vi "报告打印.vi"(9 "输出簇":T1, 11 "打印?":bool) -> ()   [LabVIEW 2010]
uses:
  <vilib>/Utility/NIReport.llb/NI_report.lvclass
  <vilib>/Utility/NIReport.llb/Append Report Text (str wrap).vi
  全局量/试验配置信息.vi
  <vilib>/addons/_office/word.llb/Word Easy Table (str).vi
  <vilib>/addons/_office/NI_ReportGenerationToolkit.lvlib
panel:
  in  "序号":i32
  out "XY图":cluster{"Y":dbl[], "Y":dbl[]}[](graph)
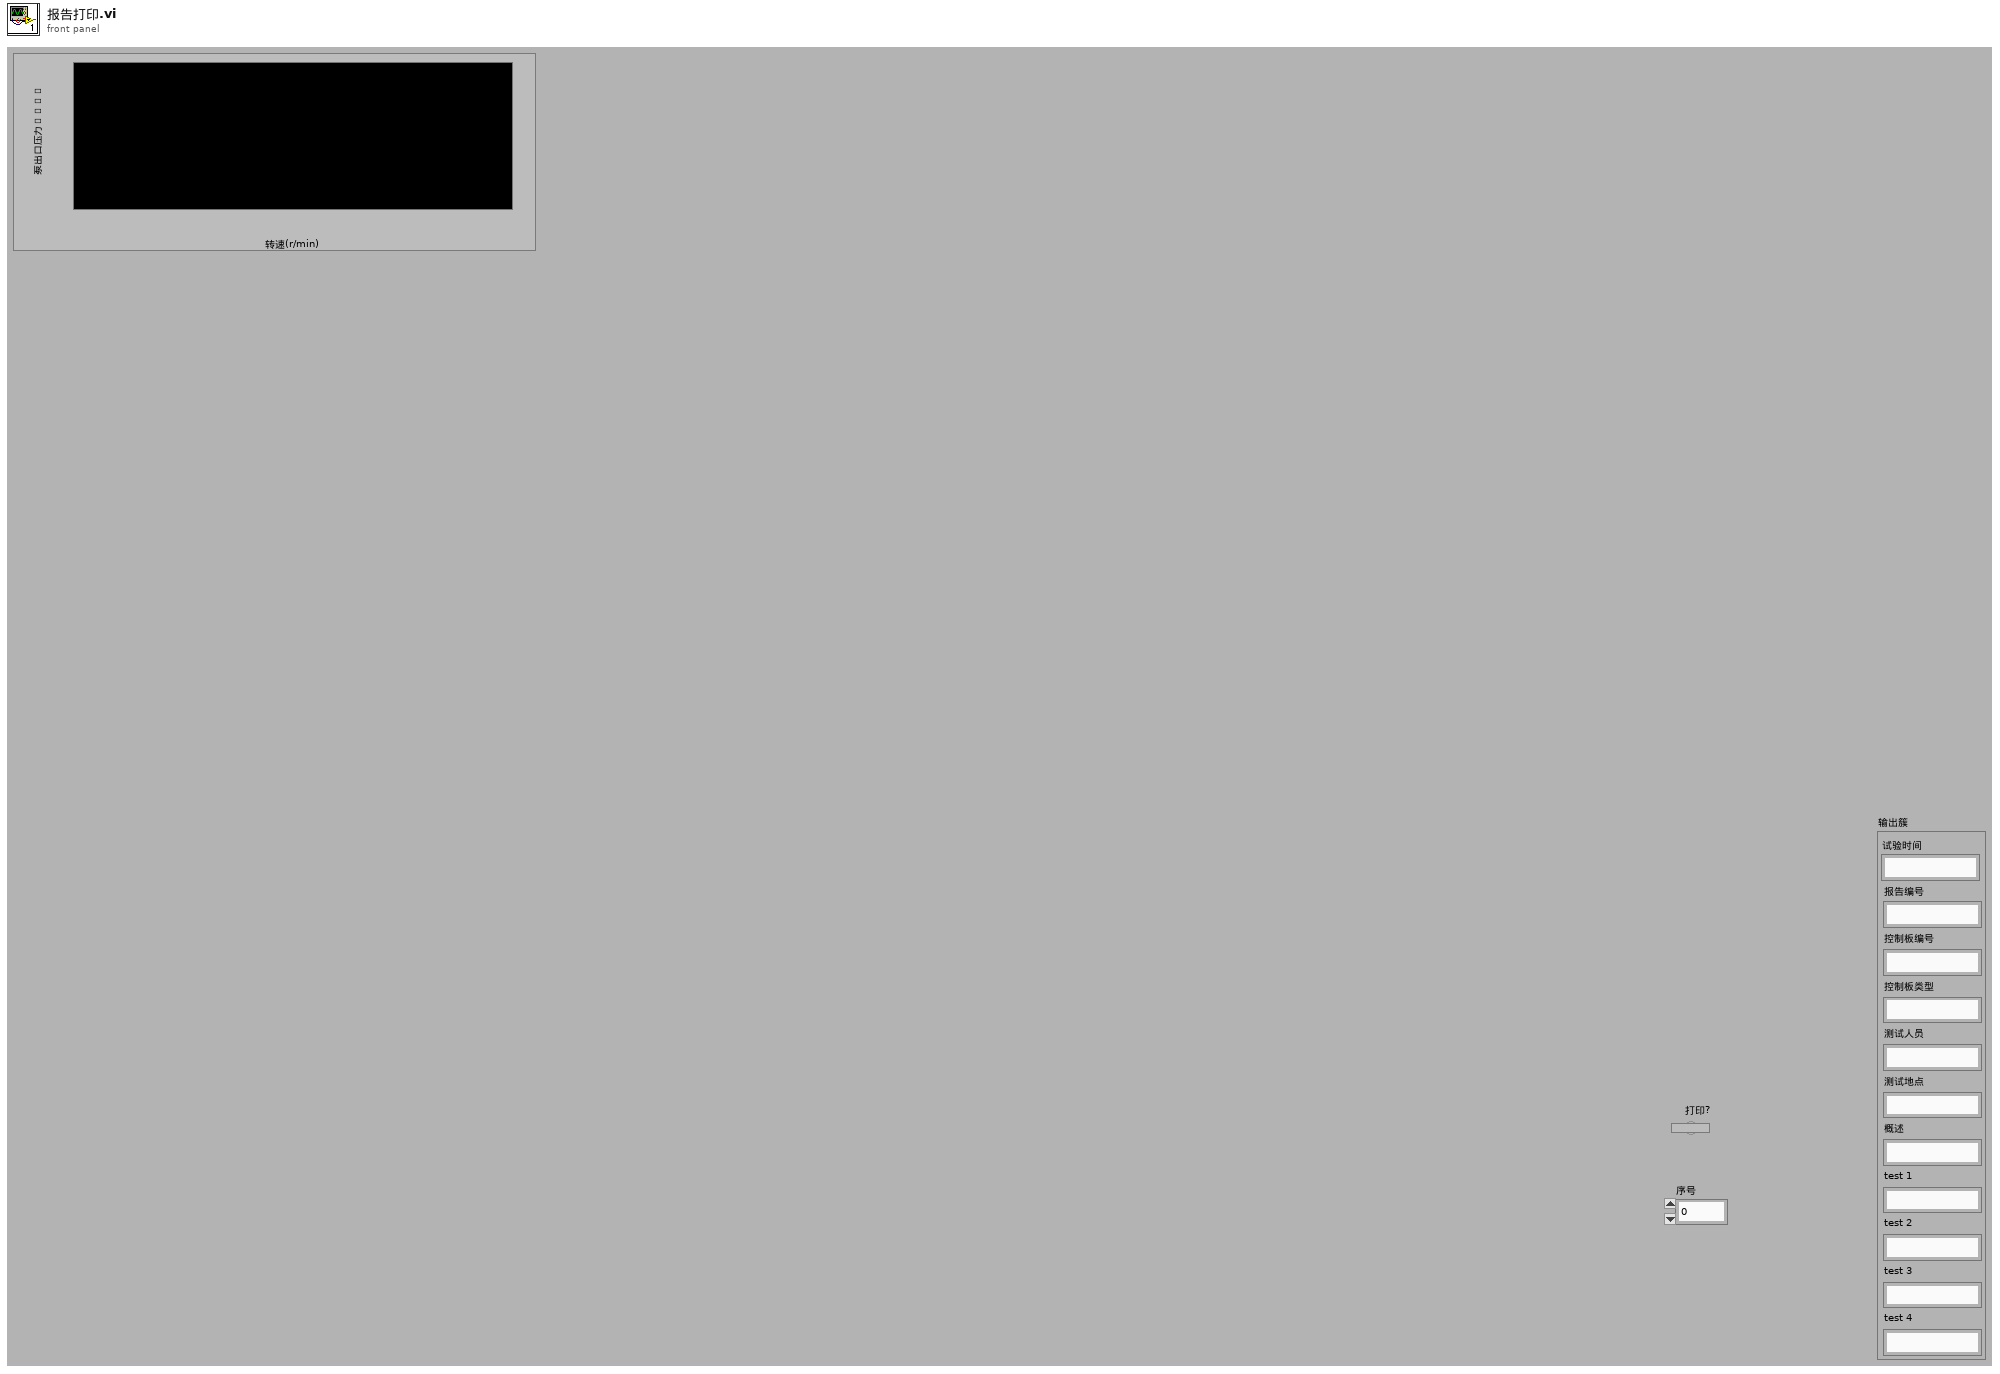
[diagram p1: front panel]
types:
  T1 = cluster{"试验时间":string, "报告编号":string, "控制板编号":string, "控制板类型":string, "测试人员":string, "测试地点":string, "概述":string, "test 1":string, "test 2":string, "test 3":string, "test 4":string}
  T2 = cluster{"position (Excel)":cluster{"row":i32, "column":i32}, "name (Excel)":string, "bookmark (Word)":string}
  T3 = enum16{"maximized", "minimized", "normal", "no change"}
  T4 = enum16{"Standard Report", "HTML", "Word", "Excel"}
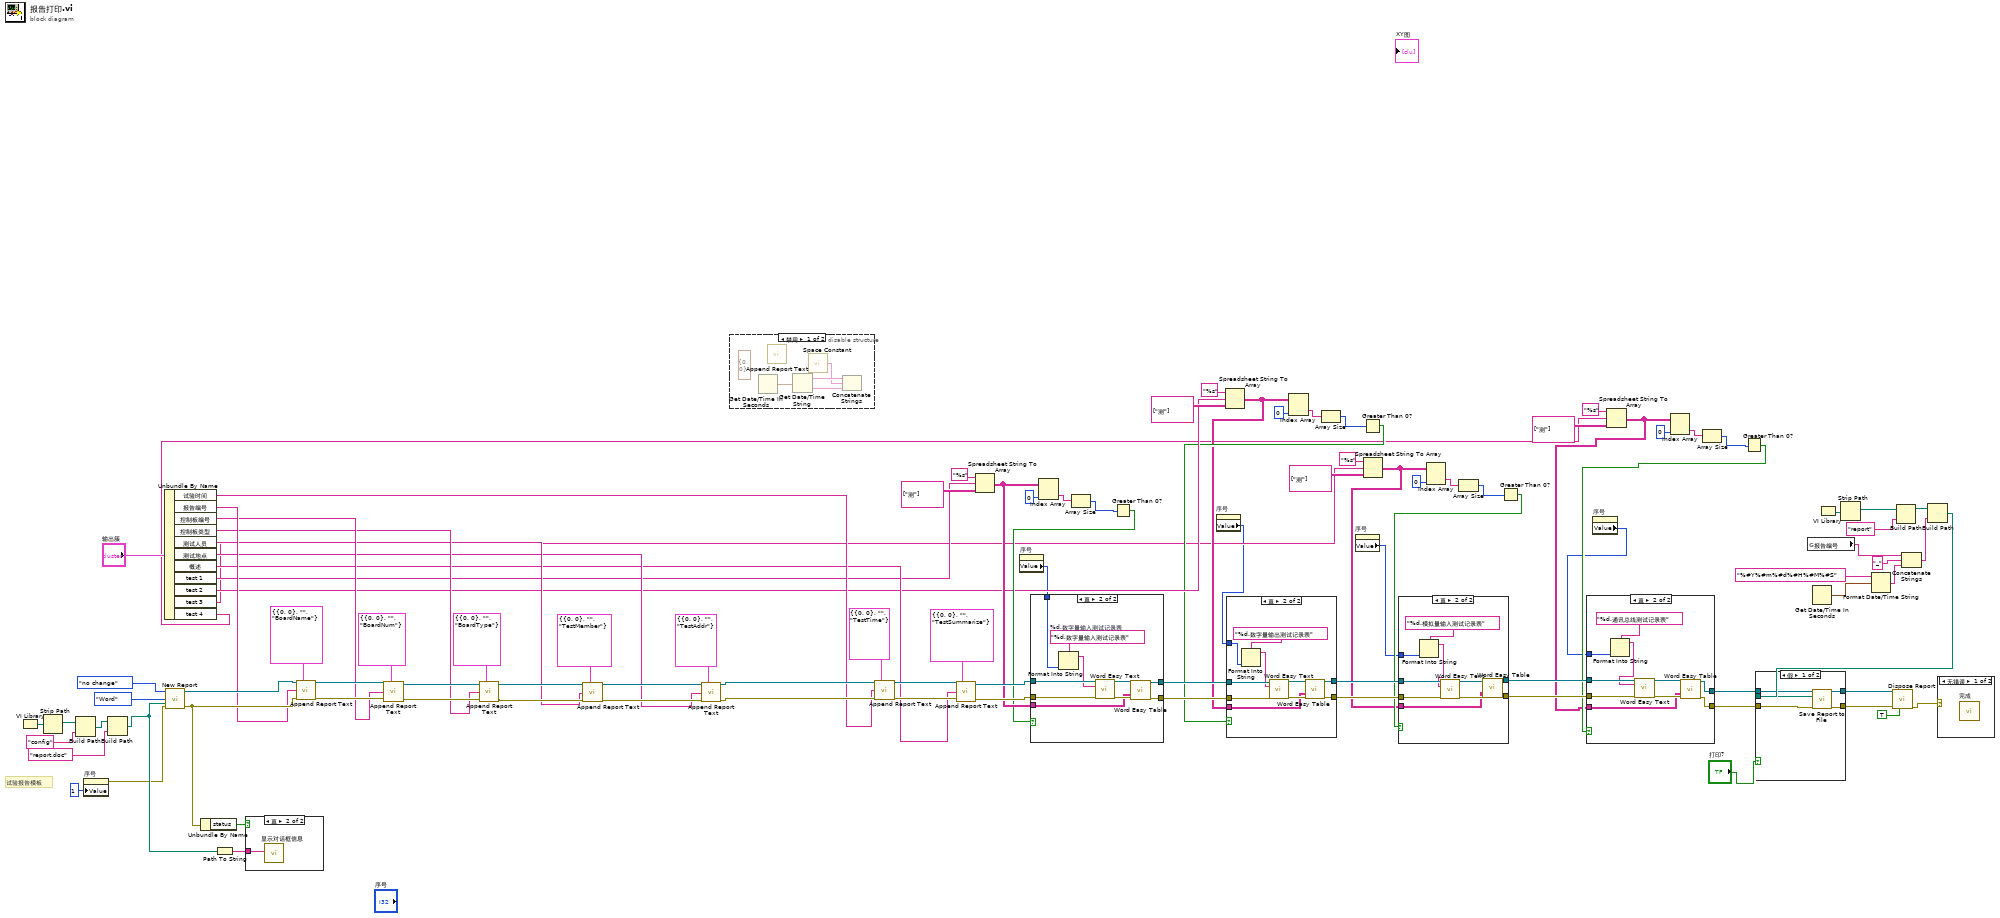
[diagram p0: block diagram]
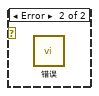
[diagram p6: hidden frame]
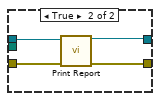
[diagram p7: hidden frame]
diagram:
  # "试验报告模板"
  n1 = VI Library() -> (path=w97:path)
  n2 = Strip Path(path=w97) -> (stripped path=w94:path)  [unwired: 1 out]
  n3 = Build Path(base path=w94, name or relative path="config") -> (appended path=w96:path)
  n4 = property on="序号" class="DigNum (严格)"("Value"=1 ("序号")) -> (error out=w49:errorcluster)  [unwired: 2 in, 1 out]
  n5 = Build Path(base path=w96, name or relative path="report.doc") -> (appended path=w100:path)
  n6 = Unbundle By Name("输出簇") -> ("试验时间"=w39:string, "报告编号"=w44:string, "控制板编号"=w43:string, "控制板类型"=w42:string, "测试人员"=w41:string, "测试地点"=w40:string, "概述"=w38:string, "test 1"=w35:string, "test 2"=w25:string, "test 3"=w18:string, "test 4"=w11:string)
  n7 = call <vilib>:"New Report.vi"("window state (normal)"=T3."no change", "report type"=T4."Word", "template (empty)"=w100, "error in (no error)"=w49) -> ("report out"=w91:refnum<class "NI_report.lvclass">, "error out"=w90:errorcluster)  [unwired: 10 in]
  n8 = Unbundle By Name(w90) -> ("status"=w102:bool)
  n9 = Path To String(path=w100) -> (string=w101:string)
  n10 = case shown="真" w102 {
    tunnel: w101 -> [_ w104]
    frame False {
    }
    frame True {
      n11 = call "显示对话框信息"("Message"=w104) -> ()  [unwired: 9 in, 2 out]
    }
  }
  n12 = call-poly <vilib>:"Append Report Text.vi"("report in"=w91, "MS Office parameters"=T2 {"position (Excel)"={"row"=0, "column"=0}, "name (Excel)"="", "bookmark (Word)"="BoardName"}, "text"=w44, "error in (no error)"=w90) -> ("report out"=w76:refnum<class "NI_report.lvclass">, "error out"=w75:errorcluster)  [unwired: 8 in, 2 out]
  n13 = call-poly <vilib>:"Append Report Text.vi"("report in"=w76, "MS Office parameters"=T2 {"position (Excel)"={"row"=0, "column"=0}, "name (Excel)"="", "bookmark (Word)"="BoardNum"}, "text"=w43, "error in (no error)"=w75) -> ("report out"=w86:refnum<class "NI_report.lvclass">, "error out"=w85:errorcluster)  [unwired: 8 in, 2 out]
  n14 = call-poly <vilib>:"Append Report Text.vi"("report in"=w86, "MS Office parameters"=T2 {"position (Excel)"={"row"=0, "column"=0}, "name (Excel)"="", "bookmark (Word)"="BoardType"}, "text"=w42, "error in (no error)"=w85) -> ("report out"=w83:refnum<class "NI_report.lvclass">, "error out"=w82:errorcluster)  [unwired: 8 in, 2 out]
  n15 = call-poly <vilib>:"Append Report Text.vi"("report in"=w83, "MS Office parameters"=T2 {"position (Excel)"={"row"=0, "column"=0}, "name (Excel)"="", "bookmark (Word)"="TestMember"}, "text"=w41, "error in (no error)"=w82) -> ("report out"=w80:refnum<class "NI_report.lvclass">, "error out"=w79:errorcluster)  [unwired: 8 in, 2 out]
  n16 = call-poly <vilib>:"Append Report Text.vi"("report in"=w80, "MS Office parameters"=T2 {"position (Excel)"={"row"=0, "column"=0}, "name (Excel)"="", "bookmark (Word)"="TestAddr"}, "text"=w40, "error in (no error)"=w79) -> ("report out"=w78:refnum<class "NI_report.lvclass">, "error out"=w77:errorcluster)  [unwired: 8 in, 2 out]
  n17 = disable-structure shown="禁用" {
    frame Disabled {
      (unwired) cluster{"row":i32, "column":i32} {"row"=0, "column"=0} ("position (excel)")
      n18 = Get Date/Time In Seconds() -> (seconds since 1Jan1904=w108:timestamp)
      n19 = call-poly <vilib>:"Append Report Text.vi"() -> ()  [unwired: 12 in, 4 out]
      n20 = Get Date/Time String(seconds (now)=w108) -> (date string=w107:string, time string=w106:string)  [unwired: 2 in]
      n21 = call <vilib>:"Space Constant.vi"() -> ("String"=w105:string)
      n22 = Concatenate Strings(w107, w105, w106) -> ()  [unwired: 1 out]
    }
    frame Enabled {
    }
  }
  n23 = call-poly <vilib>:"Append Report Text.vi"("report in"=w78, "MS Office parameters"=T2 {"position (Excel)"={"row"=0, "column"=0}, "name (Excel)"="", "bookmark (Word)"="TestTime"}, "text"=w39, "error in (no error)"=w77) -> ("report out"=w54:refnum<class "NI_report.lvclass">, "error out"=w53:errorcluster)  [unwired: 8 in, 2 out]
  n24 = call-poly <vilib>:"Append Report Text.vi"("report in"=w54, "MS Office parameters"=T2 {"position (Excel)"={"row"=0, "column"=0}, "name (Excel)"="", "bookmark (Word)"="TestSummarize"}, "text"=w38, "error in (no error)"=w53) -> ("report out"=w52:refnum<class "NI_report.lvclass">, "error out"=w51:errorcluster)  [unwired: 8 in, 2 out]
  n25 = Spreadsheet String To Array(format string="%s" ("格式字符串"), spreadsheet string=w35, array type (2D Dbl)=string[][] [["测"]] ("数组类型(2D String)")) -> (array=w34:string[][])  [unwired: 1 in]
  n26 = property on="序号" class="DigNum (严格)"() -> ("Value"=w7:i32)  [unwired: 2 in, 2 out]
  n27 = Index Array(array=w34, index (col)=0 ("禁用的索引 (列)")) -> (element=w32:string[])  [unwired: 1 in]
  n28 = Array Size(array=w32) -> (size(s)=w31:i32)
  n29 = Greater Than 0?(x=w31) -> (x > 0?=w30:bool)
  n30 = case shown="真" w30 {
    tunnel: [w110 w119] -> w61
    tunnel: [w109 w118] -> w59
    tunnel: w52 -> [w110 w116]
    tunnel: w51 -> [w109 w115]
    tunnel: w34 -> [_ w112]
    tunnel: w7 -> [_ w111]
    frame False {
    }
    frame True {
      w114 = "%d.数字量输入测试记录表"  # %d.数字量输入测试记录表
      n31 = Format Into String(format string=w114, w111) -> (resulting string=w113:string)  [unwired: 2 in, 1 out]
      n32 = call <vilib>:"Word Easy Text.vi"("report in"=w116, "text"=w113, "error in (no error)"=w115) -> ("report out"=w120:refnum<class "NI_report.lvclass">, "error out"=w117:errorcluster)  [unwired: 10 in, 1 out]
      n33 = call-poly <vilib>:"Word Easy Table.vi"("report in"=w120, "data"=w112, "error in (no error)"=w117) -> ("report out"=w119:refnum<class "NI_report.lvclass">, "error out"=w118:errorcluster)  [unwired: 10 in, 1 out]
    }
  }
  n34 = property on="序号" class="DigNum (严格)"() -> ("Value"=w6:i32)  [unwired: 2 in, 2 out]
  n35 = Spreadsheet String To Array(format string="%s" ("格式字符串"), spreadsheet string=w25, array type (2D Dbl)=string[][] [["测"]] ("数组类型(2D String)")) -> (array=w23:string[][])  [unwired: 1 in]
  n36 = Index Array(array=w23, index (col)=0 ("禁用的索引 (列)")) -> (element=w26:string[])  [unwired: 1 in]
  n37 = Array Size(array=w26) -> (size(s)=w5:i32)
  n38 = property on="序号" class="DigNum (严格)"() -> ("Value"=w4:i32)  [unwired: 2 in, 2 out]
  n39 = Greater Than 0?(x=w5) -> (x > 0?=w24:bool)
  n40 = case shown="真" w24 {
    tunnel: w61 -> [w122 w132]
    tunnel: [w122 w130] -> w60
    tunnel: w59 -> [w121 w129]
    tunnel: [w121 w127] -> w58
    tunnel: w6 -> [_ w124]
    tunnel: w23 -> [_ w123]
    frame False {
    }
    frame True {
      n41 = Format Into String(format string="%d.数字量输出测试记录表", w124) -> (resulting string=w125:string)  [unwired: 2 in, 1 out]
      n42 = call <vilib>:"Word Easy Text.vi"("report in"=w132, "text"=w125, "error in (no error)"=w129) -> ("report out"=w131:refnum<class "NI_report.lvclass">, "error out"=w128:errorcluster)  [unwired: 10 in, 1 out]
      n43 = call-poly <vilib>:"Word Easy Table.vi"("report in"=w131, "data"=w123, "error in (no error)"=w128) -> ("report out"=w130:refnum<class "NI_report.lvclass">, "error out"=w127:errorcluster)  [unwired: 10 in, 1 out]
    }
  }
  n44 = Spreadsheet String To Array(format string="%s" ("格式字符串"), spreadsheet string=w18, array type (2D Dbl)=string[][] [["测"]] ("数组类型(2D String)")) -> (array=w16:string[][])  [unwired: 1 in]
  n45 = Index Array(array=w16, index (col)=0 ("禁用的索引 (列)")) -> (element=w19:string[])  [unwired: 1 in]
  n46 = Array Size(array=w19) -> (size(s)=w3:i32)
  n47 = Greater Than 0?(x=w3) -> (x > 0?=w17:bool)
  n48 = case shown="真" w17 {
    tunnel: w60 -> [w134 w144]
    tunnel: w58 -> [w133 w142]
    tunnel: [w134 w140] -> w57
    tunnel: [w133 w139] -> w56
    tunnel: w4 -> [_ w136]
    tunnel: w16 -> [_ w135]
    frame False {
    }
    frame True {
      n49 = Format Into String(format string="%d.模拟量输入测试记录表", w136) -> (resulting string=w137:string)  [unwired: 2 in, 1 out]
      n50 = call <vilib>:"Word Easy Text.vi"("report in"=w144, "text"=w137, "error in (no error)"=w142) -> ("report out"=w143:refnum<class "NI_report.lvclass">, "error out"=w141:errorcluster)  [unwired: 10 in, 1 out]
      n51 = call-poly <vilib>:"Word Easy Table.vi"("report in"=w143, "data"=w135, "error in (no error)"=w141) -> ("report out"=w140:refnum<class "NI_report.lvclass">, "error out"=w139:errorcluster)  [unwired: 10 in, 1 out]
    }
  }
  n52 = property on="序号" class="DigNum (严格)"() -> ("Value"=w2:i32)  [unwired: 2 in, 2 out]
  n53 = Spreadsheet String To Array(format string="%s" ("格式字符串"), spreadsheet string=w11, array type (2D Dbl)=string[][] [["测"]] ("数组类型(2D String)")) -> (array=w9:string[][])  [unwired: 1 in]
  n54 = Index Array(array=w9, index (col)=0 ("禁用的索引 (列)")) -> (element=w12:string[])  [unwired: 1 in]
  n55 = Array Size(array=w12) -> (size(s)=w1:i32)
  n56 = Greater Than 0?(x=w1) -> (x > 0?=w10:bool)
  n57 = case shown="真" w10 {
    tunnel: [w146 w156] -> w63
    tunnel: [w145 w155] -> w62
    tunnel: w57 -> [w146 w154]
    tunnel: w56 -> [w145 w153]
    tunnel: w2 -> [_ w148]
    tunnel: w9 -> [_ w147]
    frame False {
    }
    frame True {
      n58 = Format Into String(format string="%d.通讯总线测试记录表", w148) -> (resulting string=w149:string)  [unwired: 2 in, 1 out]
      n59 = call <vilib>:"Word Easy Text.vi"("report in"=w154, "text"=w149, "error in (no error)"=w153) -> ("report out"=w152:refnum<class "NI_report.lvclass">, "error out"=w151:errorcluster)  [unwired: 10 in, 1 out]
      n60 = call-poly <vilib>:"Word Easy Table.vi"("report in"=w152, "data"=w147, "error in (no error)"=w151) -> ("report out"=w156:refnum<class "NI_report.lvclass">, "error out"=w155:errorcluster)  [unwired: 10 in, 1 out]
    }
  }
  n61 = global read "试验配置信息.vi" "报告编号"() -> (w47:string)
  n62 = Get Date/Time In Seconds() -> (seconds since 1Jan1904=w69:timestamp)
  n63 = VI Library() -> (path=w70:path)
  n64 = Strip Path(path=w70) -> (stripped path=w73:path)  [unwired: 1 out]
  n65 = Format Date/Time String(time format string (%c)="%#Y%#m%#d%#H%#M%#S" ("时间格式字符串(%c)"), seconds (now)=w69) -> (date/time string=w48:string)  [unwired: 1 in]
  n66 = Build Path(base path=w73, name or relative path="report") -> (appended path=w71:path)
  n67 = Concatenate Strings(w47, "_", w48) -> (w45:string)
  n68 = Build Path(base path=w71, name or relative path=w45) -> (appended path=w65:path)
  n69 = case shown="假" "打印?" {
    tunnel: w63 -> [w161 w165]
    tunnel: w62 -> [w160 w164]
    tunnel: [w159 w163] -> w67
    tunnel: [w158 w162] -> w66
    tunnel: w65 -> [w157 _]
    frame False {
      n70 = call-dynamic "Save Report to File.vi"("report in"=w161, "report file path"=w157, "error in (no error)"=w160) -> ("report out"=w159:refnum<class "NI_report.lvclass">, "error out"=w158:errorcluster)  [unwired: 11 in]
    }
    frame True {
      n71 = call-dynamic "Print Report.vi"("report in"=w165, "error in (no error)"=w164) -> ("report out"=w163:refnum<class "NI_report.lvclass">, "error out"=w162:errorcluster)  [unwired: 12 in]
    }
  }
  n72 = call-dynamic "Dispose Report.vi"("report in"=w67, "error in (no error)"=w66, "close report? (T)"=TRUE) -> ("error out"=w64:errorcluster)  [unwired: 12 in]
  n73 = case shown="无错误" w64 {
    frame No Error {
      n74 = call "完成"() -> ()  [unwired: 10 in, 2 out]
    }
    frame Error {
      n75 = call "错误"() -> ()  [unwired: 10 in, 2 out]
    }
  }
